vi "zeros-padded-color (SubVI).vi"(9 "Value":u8, 10 "image data":T1, 11 "Array":u8[](array[numeric])) -> (3 "Real Matrix":T2)   [LabVIEW 2015]
uses:
  <vilib>/Analysis/Matrix/Datatypes/RealMatrix.ctl
  <vilib>/Analysis/Matrix/NI_Matrix.lvlib
  <vilib>/picture/picture.llb/imagedata.ctl
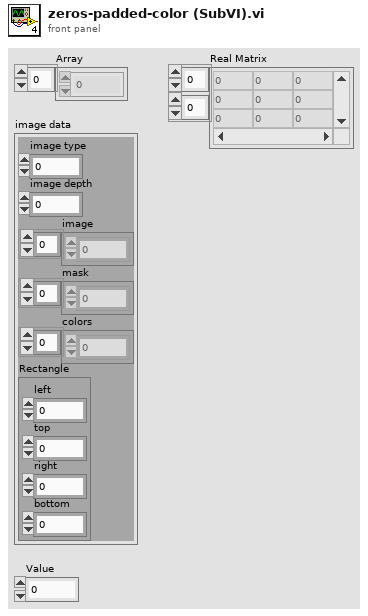
[diagram p1: front panel]
types:
  T1 = typedef "imagedata.ctl" = cluster{"image type":i32, "image depth":i32, "image":u8[], "mask":u8[], "colors":u32[], "Rectangle":cluster{"left":i16, "top":i16, "right":i16, "bottom":i16}}
  T2 = typedef "NI_Matrix.lvlib/RealMatrix.ctl" = dbl[][]
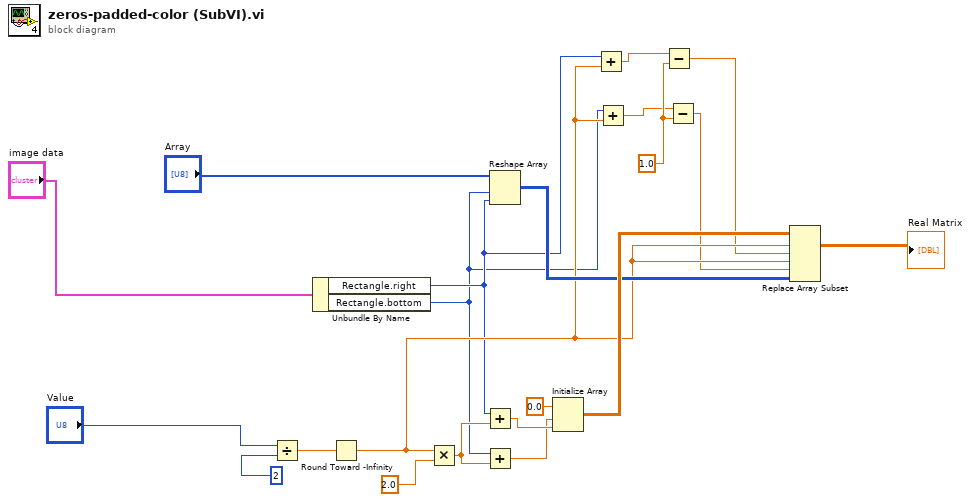
[diagram p0: block diagram]
diagram:
  w8 = 1.0 ("y")
  n1 = Divide(x="Value", y=u8 2) -> (x/y=w9:dbl)
  n2 = Unbundle By Name("image data") -> ("Rectangle.right"=w4:i16, "Rectangle.bottom"=w3:i16)
  n3 = Round Toward -Infinity(1:w9) -> (0:w5:dbl)
  n4 = Multiply(x=w5, y=2.0) -> (x*y=w15:dbl)
  n5 = Add(x=w4, y=w15) -> (x+y=w20:dbl)
  n6 = Add(x=w3, y=w15) -> (x+y=w19:dbl)
  n7 = Reshape Array("Array", w3, w4) -> (w17:u8[][])
  n8 = Initialize Array(0.0 ("element"), w19, w20) -> (w18:dbl[][])
  n9 = Add(x=w4, y=w5) -> (x+y=w7:dbl)
  n10 = Add(x=w3, y=w5) -> (x+y=w6:dbl)
  n11 = Subtract(x=w7, y=w8) -> (x-y=w2:dbl)
  n12 = Subtract(x=w6, y=w8) -> (x-y=w1:dbl)
  n13 = Replace Array Subset(array=w18, new element=w17, index (dim 0)=w5, index (dim 1)=w2, index (dim 2)=w5, index (dim 3)=w1) -> (→"Real Matrix":T2)
